vi "AVL GNU umrechnen ALST.vi"(10 "Konzentration":dbl, 11 "Teilerstufe in%":string) -> (3 "Konzentration":string)   [LabVIEW 2020, in "Linearisierung v2.lvlib" / "Gasteiler.lvlib"]
uses:
  Gasteiler.lvlib
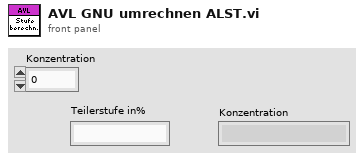
[diagram p1: front panel]
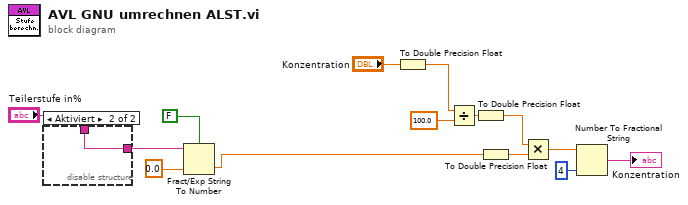
[diagram p0: block diagram]
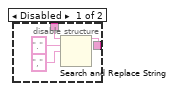
[diagram p2: hidden frame]
diagram:
  n1 = disable-structure shown="Aktiviert" {
    disable-tunnel: "Teilerstufe in%" -> [w16 w19]
    disable-tunnel: [w15 w19] -> w7
    frame Disabled {
      n2 = Search and Replace String(input string=w16, search string="." ("Such-String"), replace string="," ("String ersetzen(\"\")")) -> (result string=w15:string)  [unwired: 5 in, 3 out]
    }
    frame Enabled {
    }
  }
  n3 = Fract/Exp String To Number(use system decimal point (T)=FALSE ("Systemdezimalzeichen verwenden (T)"), string=w7, default (0 dbl)=sgl 0.0) -> (number=w3:sgl)  [unwired: 1 in, 1 out]
  n4 = To Double Precision Float(number="Konzentration") -> (double precision float=w2:dbl)
  n5 = Divide(x=w2, y=100.0) -> (x/y=w12:dbl)
  n6 = To Double Precision Float(number=w12) -> (double precision float=w6:dbl)
  n7 = To Double Precision Float(number=w3) -> (double precision float=w5:dbl)
  n8 = Multiply(x=w6, y=w5) -> (x*y=w4:dbl)
  n9 = Number To Fractional String(number=w4, precision (6)=i16 4 ("Genauigkeit (6)")) -> (F-format string=→"Konzentration":string)  [unwired: 2 in]
